vi "Drive Write Test(SubVI).vi"   [LabVIEW 2014]
uses:
  Global Variables/Sensor Data (Edited).vi
  <vilib>/Rock Robotics/Network Tables/SD Write Number.vi
  <vilib>/Rock Robotics/Network Tables/SD Write Numeric Array.vi
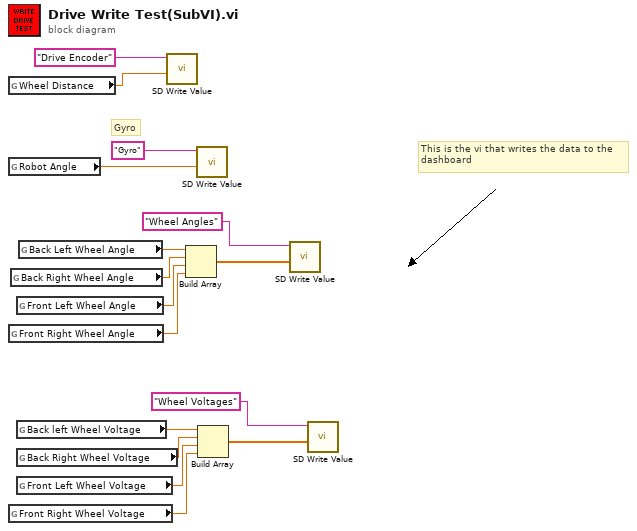
[diagram p0: block diagram]
diagram:
  # "This is the vi that writes the data to the \ndashboard"
  # "Gyro"
  n1 = global read "Sensor Data (Edited).vi" "Wheel Distance"() -> (w15:dbl)
  n2 = global read "Sensor Data (Edited).vi" "Robot Angle"() -> (w13:dbl)
  n3 = global read "Sensor Data (Edited).vi" "Front Right Wheel Angle"() -> (w9:dbl)
  n4 = global read "Sensor Data (Edited).vi" "Front Right Wheel Voltage"() -> (w3:dbl)
  n5 = global read "Sensor Data (Edited).vi" "Back Right Wheel Angle"() -> (w11:dbl)
  n6 = global read "Sensor Data (Edited).vi" "Front Left Wheel Angle"() -> (w10:dbl)
  n7 = global read "Sensor Data (Edited).vi" "Back left Wheel Voltage"() -> (w6:dbl)
  n8 = global read "Sensor Data (Edited).vi" "Back Right Wheel Voltage"() -> (w5:dbl)
  n9 = global read "Sensor Data (Edited).vi" "Front Left Wheel Voltage"() -> (w4:dbl)
  n10 = global read "Sensor Data (Edited).vi" "Back Left Wheel Angle"() -> (w12:dbl)
  n11 = call-poly <vilib>:"SD Write Value.vi"("Numeric"=w15, "Name"="Drive Encoder") -> ()  [unwired: 8 in, 2 out]
  n12 = Build Array(w12, w11, w10, w9) -> (w8:dbl[])
  n13 = call-poly <vilib>:"SD Write Value.vi"("Numeric"=w13, "Name"="Gyro") -> ()  [unwired: 8 in, 2 out]
  n14 = Build Array(w6, w5, w4, w3) -> (w2:dbl[])
  n15 = call-poly <vilib>:"SD Write Value.vi"("Numeric Array"=w8, "Name"="Wheel Angles") -> ()  [unwired: 8 in, 2 out]
  n16 = call-poly <vilib>:"SD Write Value.vi"("Numeric Array"=w2, "Name"="Wheel Voltages") -> ()  [unwired: 8 in, 2 out]
